vi "Sequence Error Log.vi"(10 "string":string, 11 "Byte Stream File in":refnum<file>) -> ()   [LabVIEW 2018, in "Sequencing Library.lvlib"]
uses:
  Sequencing Library.lvlib
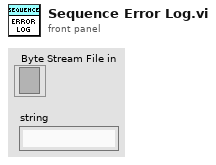
[diagram p1: front panel]
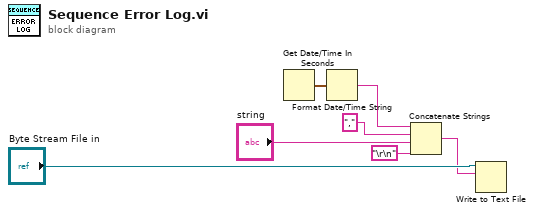
[diagram p0: block diagram]
diagram:
  n1 = Get Date/Time In Seconds() -> (seconds since 1Jan1904=w2:timestamp)
  n2 = Format Date/Time String(seconds (now)=w2) -> (date/time string=w1:string)  [unwired: 2 in]
  n3 = Concatenate Strings(w1, "," ("string"), "string", "\r\n") -> (w3:string)
  n4 = Write to Text File(file (use dialog)="Byte Stream File in", text=w3) -> ()  [unwired: 2 in, 3 out]
